vi "isForEditing.vi"(8 "error in (no error)":errorcluster, 11 "ActionPanel in":refnum<class "ActionPanel.lvclass">) -> (0 "error out":errorcluster, 2 "editing?":bool, 3 "ActionPanel out":refnum<class "ActionPanel.lvclass">)   [LabVIEW 2009, in "Views.lvlib" / "ScriptEditor.lvlib" / "ActionPanel.lvclass"]
uses:
  ActionPanel.lvclass
  Tools/Scripting/ScriptingEvent/ScriptEvent.lvclass
  ActionPanel.lvclass/ActionPanel.ctl
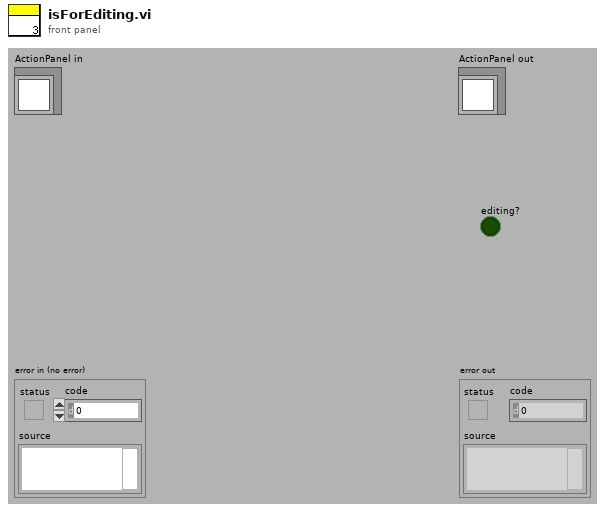
[diagram p1: front panel]
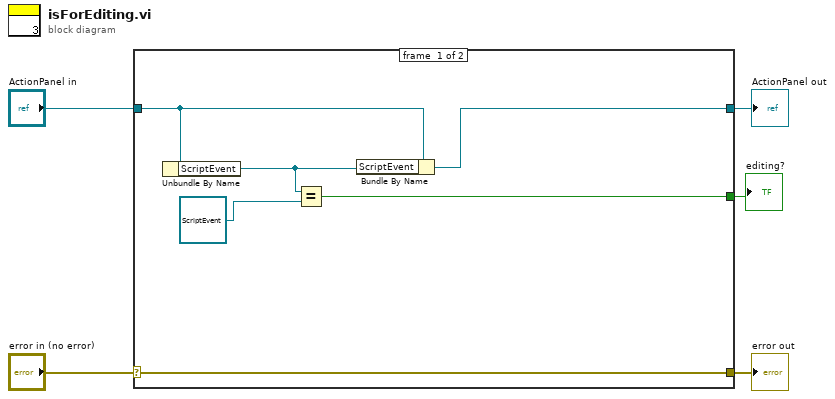
[diagram p0: block diagram]
diagram:
  n1 = case shown="No Error" "error in (no error)" {
    selector: "error in (no error)" -> [w11 w13]
    tunnel: [w11 w13] -> w4
    tunnel: [w6 w12] -> w2
    tunnel: "ActionPanel in" -> [w7 w12]
    tunnel: [w9 _] -> w1
    frame #0 {
      n2 = Unbundle By Name(w7) -> ("ScriptEvent"=w8:refnum<class "ScriptEvent.lvclass">)
      n3 = Equal?(x=w8, y=refnum<class "ScriptEvent.lvclass"> refnum ("Tools.lvlib:Scripting.lvlib:ScriptEvent.lvclass")) -> (x = y?=w9:bool)
      n4 = Bundle By Name(cluster=w7, "ScriptEvent"=w8) -> (w6:refnum<class "ActionPanel.lvclass">)
    }
    frame #1 {
    }
  }
  "error out" <- w4
  "ActionPanel out" <- w2
  "editing?" <- w1
